vi "SPI_Regs.vi"() -> (0 "Init Data Out":u8[](array[numeric]))   [LabVIEW 2018]
panel:
  in  "Регистры":u8[](array[numeric])=[35, 5, 0, 244, 1, 0, 1, 0, 0, 0, 0, 0, 34, 20, 1, 0, 0, 7, 0, 4, 0, 0, 20, 0, 0, 0, 0, 0, 0, 0, 0, 0, 0, 0, 0, 0, 0, 0, 0, 0, 0, 0, 0, 0, 0, 0, 0, 0, 0, 0, 0, 0, 0, 0, 0, 0, 0, 0, 0, 0, 0, 0, 0, 0, 0, 0, 0, 0, 0, 0, 0, 0, 0, 0, 0, 0, 0, 0, 0, 0, 0, 0, 0, 50, 20, 0, 0, 6, 2, 2, 4, 4, 0, 32, 35, 1, 196, 53, 203, 59, 53, 252, 255, 255, 255, 255, 255, 255, 255, 255, 52, 216, 16, 79, 61, 0, 8, 144, 192, 29, 9, 196, 50, 75, 91, 5, 208, 160, 195, 68, 2, 16, 112, 67, 14, 48, 208, 240, 208, 68, 7, 208, 192, 195, 68, 52, 240, 128, 195, 255, 75, 164, 161, 64, 14, 65, 252, 31, 129, 12, 124, 0, 24, 27, 1, 0, 2, 0, 5, 0, 0, 0, 7, 208, 192, 195, 68, 0, 1, 3, 0, 0, 0, 0, 0, 0, 0, 0, 0, 0, 0, 0, 0, 0, 0, 0, 0, 0, 0, 0, 0, 0, 176, 0, 27, 33, 128, 247, 131, 128, 133, 204, 119, 243, 221, 13, 211, 0, 0, 28, 176, 13, 254, 98, 193, 31, 138, 202, 231, 168, 60, 138, 254, 130, 52, 127, 193, 32, 2, 0, 0, 0, 0, 0, 0, 0, 0, 0, 0, 0, 0, 0, 0, 0, 0, 0]
  # "For Initialization VI requirements and help, please read directions located on Block Diagram."
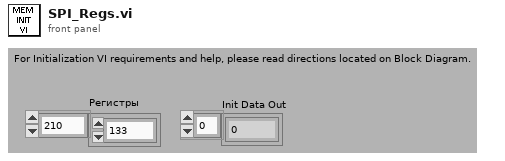
[diagram p1: front panel]
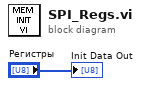
[diagram p0: block diagram]
diagram:
  "Init Data Out" <- "Регистры"
